vi "Set Encoder.vi"(8 "error in (no error)":errorcluster, 10 "encoder pos in display unit":dbl, 11 "Motor in":refnum<class "Motor.lvclass">) -> (0 "error out":errorcluster, 3 "Motor out":refnum<class "Motor.lvclass">)   [LabVIEW 2016, in "Hardware.lvlib" / "Motor.lvlib" / "Motor.lvclass"]
uses:
  <userlib>/Common Components/Hardware/Motor/Motor/Motor.lvclass
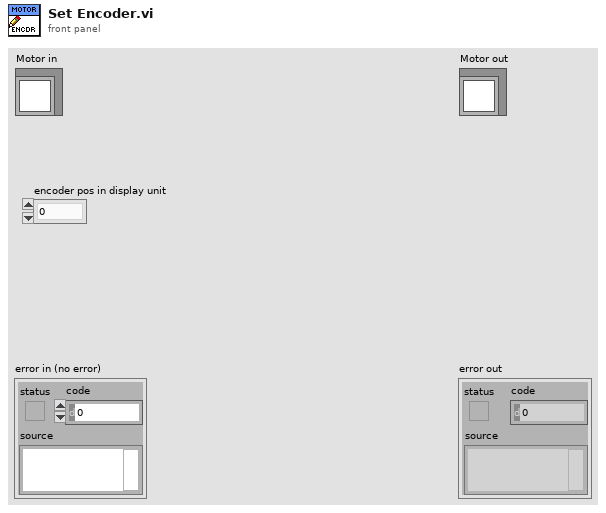
[diagram p1: front panel]
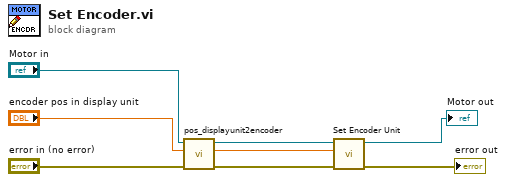
[diagram p0: block diagram]
diagram:
  n1 = call <userlib>:"pos_displayunit2encoder.vi"("error in (no error)"="error in (no error)", "pos in display unit"="encoder pos in display unit", "Motor in"="Motor in") -> ("error out"=w5:errorcluster, "encoder (unit)"=w1:dbl, "Motor out"=w3:refnum<class "Motor.lvclass">)  [unwired: 6 in]
  n2 = call-dynamic "Set Encoder Unit.vi"("error in (no error)"=w5, "encoder (unit)"=w1, "Motor in"=w3) -> ("error out"=→"error out":errorcluster, "Motor out"=→"Motor out":refnum<class "Motor.lvclass">)  [unwired: 7 in]
